vi "pxi_comms.vi"() -> ()   [LabVIEW 2017]
uses:
  <vilib>/rvi/Emulation/niFpgaGetClockAttributes.vi
  <vilib>/rvi/Emulation/niFpgaSctlEmulationGetInTimedLoop.vi
  <vilib>/rvi/Emulation/niFpgaEmulationReportErrorSimple.vi
  <vilib>/rvi/eio/common/nirviEmuTemplateMethod_errors.vi
  <vilib>/rvi/Emulation/niFpgaCriticalErrorInLSC.vi
  <vilib>/rvi/Emulation/niFpgaProcessEmulError.vi
  <vilib>/eio/EIONode/EIONode.xnode
panel:
  in  "Begin":bool
  out "Waveform Graph":i16[](graph)
  in  "Count(uSec)":u32
  in  "Numeric 5":i16
  in  "Numeric 4":i16
  in  "Numeric 3":i16
  in  "Numeric 2":i16
  in  "Numeric":i16
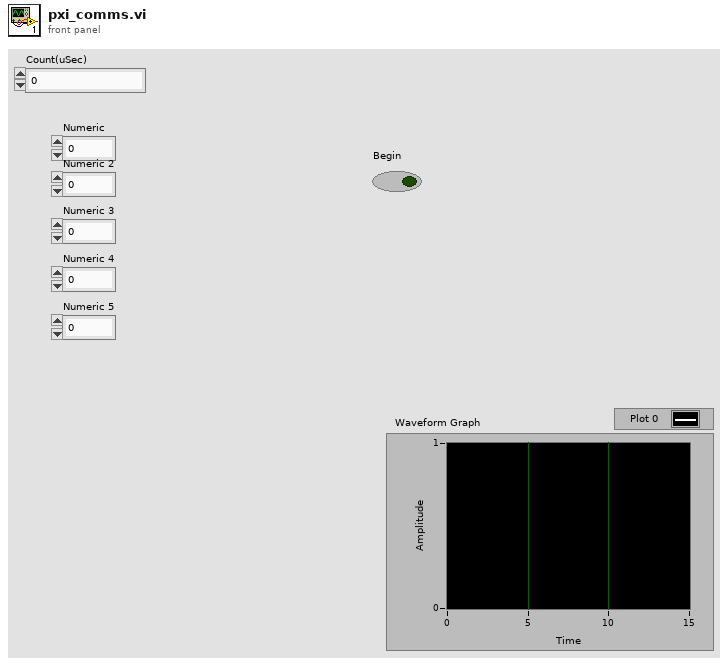
[diagram p1: front panel]
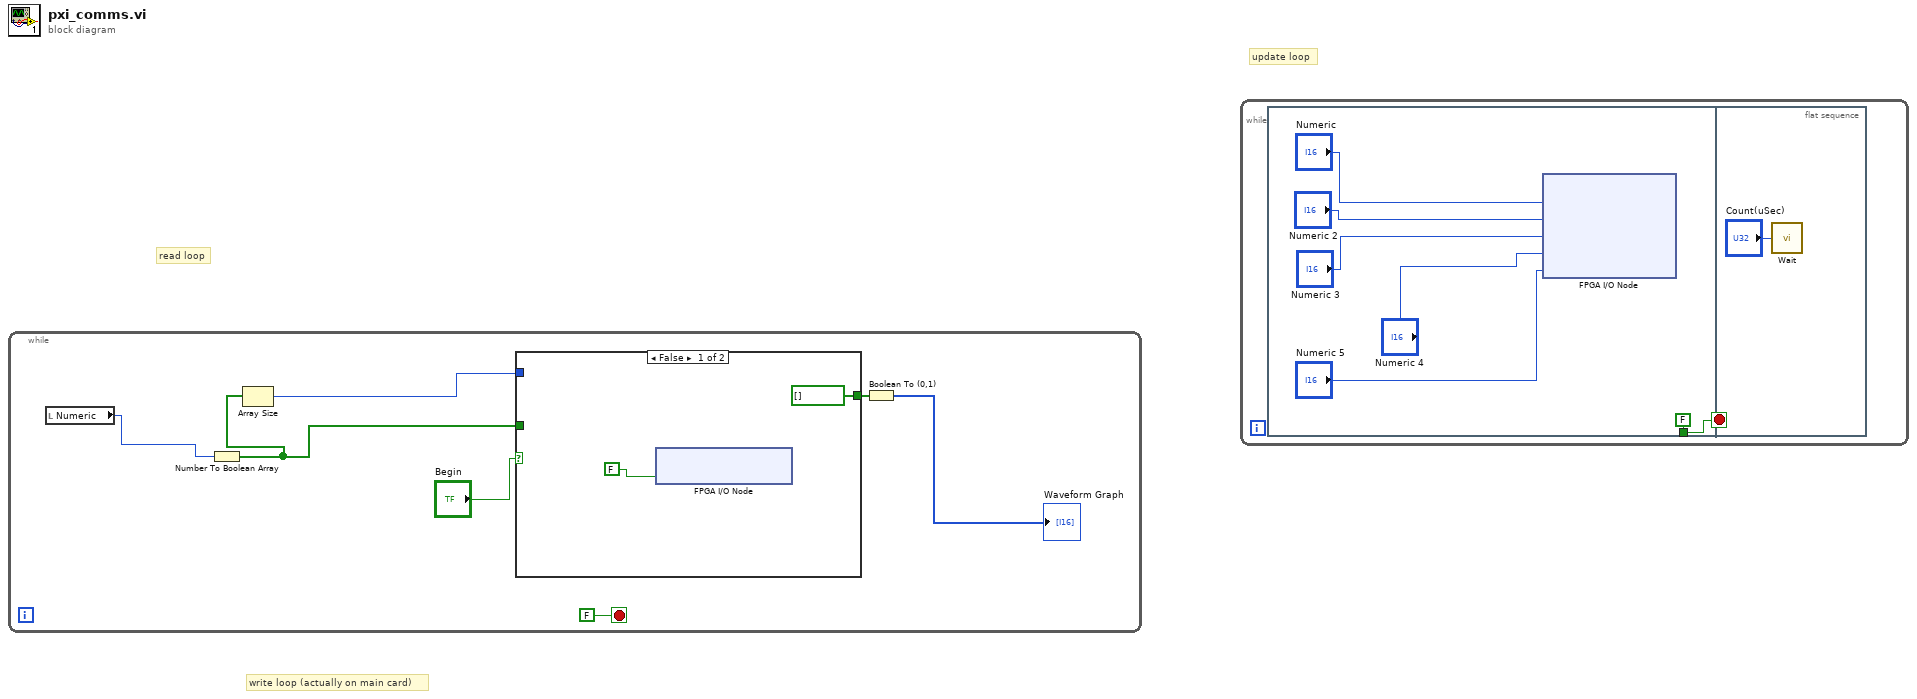
[diagram p0: block diagram]
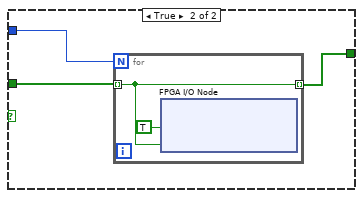
[diagram p2: hidden frame]
diagram:
  # "update loop"
  # "read loop"
  # "write loop (actually on main card)"
  n1 = while {
    stop <- FALSE stop-if-true
    n2 = local read "Numeric"() -> (w6:i16)
    n3 = Number To Boolean Array(number=w6) -> (Boolean array=w5:bool[])
    n4 = Array Size(array=w5) -> (size(s)=w4:i32)
    n5 = case shown="False" "Begin" {
      tunnel: w5 -> [_ w12]
      tunnel: w4 -> [_ w11]
      tunnel: [bool[] [] w10] -> w3
      frame False {
        n6 = xnode "FPGA I/O Node"("Connector0/DIO0"=FALSE) -> ()  [unwired: 1 in, 1 out]
      }
      frame True {
        n7 = for {
          N: w11 -> [_]
          tunnel: w12 -> [w14] mode=indexing
          tunnel: [w14] -> w10 mode=indexing
          n8 = xnode "FPGA I/O Node"("Connector0/DIO0"=TRUE, "Connector0/DIO1"=w14) -> ()  [unwired: 2 in, 2 out]
        }
      }
    }
    n9 = Boolean To (0,1)(Boolean=w3) -> (0, 1=→"Waveform Graph":i16[])
  }
  n10 = while {
    stop <- w15 stop-if-true
    n11 = flat-sequence {
      tunnel: [FALSE] -> w15
      frame #0 {
        n12 = xnode "FPGA I/O Node"("Connector0/AO0"="Numeric", "Connector0/AO1"="Numeric 2", "Connector0/AO2"="Numeric 3", "Connector0/AO3"="Numeric 4", "Connector0/AO4"="Numeric 5") -> ()  [unwired: 5 in, 5 out]
      }
      frame #1 {
        n13 = call "Wait"("Count(uSec)"="Count(uSec)") -> ()  [unwired: 1 out]
      }
    }
  }
